vi "PacketToJSON.vi"(6 "StreamType(Raw)":T1, 8 "ErrorIn":errorcluster, 10 "Packet":T2={"ID"=0, "SamplesNr"=0, "Samples"=[], "MeasurementConfig"={"Frequency"=100, "Resolution[b]"=4, "AccelFSRange"=enum."+/-2g", "GyroFSRange"=enum."+/-250dps"}, "Comment"=""} {"MeasurementConfig"."Resolution[b]" min=4 max=16 step=1; "MeasurementConfig"."Frequency" min=1 max=10000000 step=1}, 11 "JSONIn":refnum<class "JSON Object.lvclass">) -> (0 "ErrorOut":errorcluster, 2 "JSONPacket":string, 3 "JSONOut":refnum<class "JSON Object.lvclass">)   [LabVIEW 2016]
doc: "Convert Packet to JSON. Return also JSONOut to combine with other JSON objects."
uses:
  FallSensor/Packet.ctl
  FallSensor/Sample.ctl
  FallSensor/Reading.ctl
  FallSensor/MeasurementConfig.ctl
  FallSensor/Measurement/AccelFSRange.ctl
  FallSensor/Measurement/GyroFSRange.ctl
  <vilib>/addons/JSON API/JSON Object/JSON Object.lvclass
  D:/Programy/National Instruments/LabVIEW 2016/vi.lib/addons/JSON API/JSON Value/JSON Value.lvclass
  JSONStreamType.ctl
  <vilib>/addons/JSON API/JSON Object/Set Object Item by name.vi
  <vilib>/addons/JSON API/JSON Value/Get as JSON string.vi
  <vilib>/addons/JSON API/JSON Scalar/JSON Scalar.lvclass
  <vilib>/addons/JSON API/JSON Array/JSON Array.lvclass
  <vilib>/addons/JSON API/JSON Scalar/Set U32.vi
  <vilib>/addons/JSON API/JSON Scalar/Set String.vi
  <vilib>/addons/JSON API/JSON Array/Set JSON Array.vi
  <vilib>/addons/JSON API/JSON Value/Get as JSON string (pretty).vi
  <vilib>/addons/JSON API/JSON Value/Get Item by name array.vi
  <vilib>/addons/JSON API/JSON Value/JSON Value.lvclass
  <vilib>/addons/JSON API/Get Polymorphic/JSON GetSet.lvlib
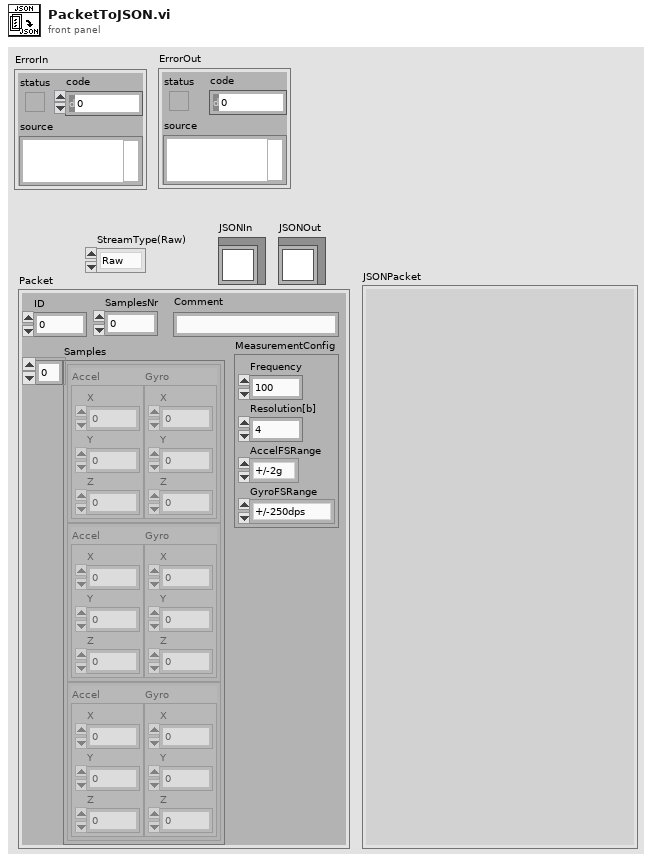
[diagram p1: front panel]
types:
  T1 = typedef "JSONStreamType.ctl" = enum16{"Raw", "Pretty"}
  T2 = typedef "Packet.ctl" = cluster{"ID":u32, "SamplesNr":u32, "Samples":T3[], "MeasurementConfig":T5, "Comment":string}
  T3 = typedef "Sample.ctl" = cluster{"Accel":T4, "Gyro":T4}
  T4 = typedef "Reading.ctl" = cluster{"X":i16, "Y":i16, "Z":i16}
  T5 = typedef "MeasurementConfig.ctl" = cluster{"Frequency":u32, "Resolution[b]":u32, "AccelFSRange":T6, "GyroFSRange":T7}
  T6 = typedef "AccelFSRange.ctl" = enum16{"+/-2g", "+/-4g", "+/-8g", "+/-16g"}
  T7 = typedef "GyroFSRange.ctl" = enum16{"+/-250dps", "+/-500dps", "+/-1000dps", "+/-2000dps"}
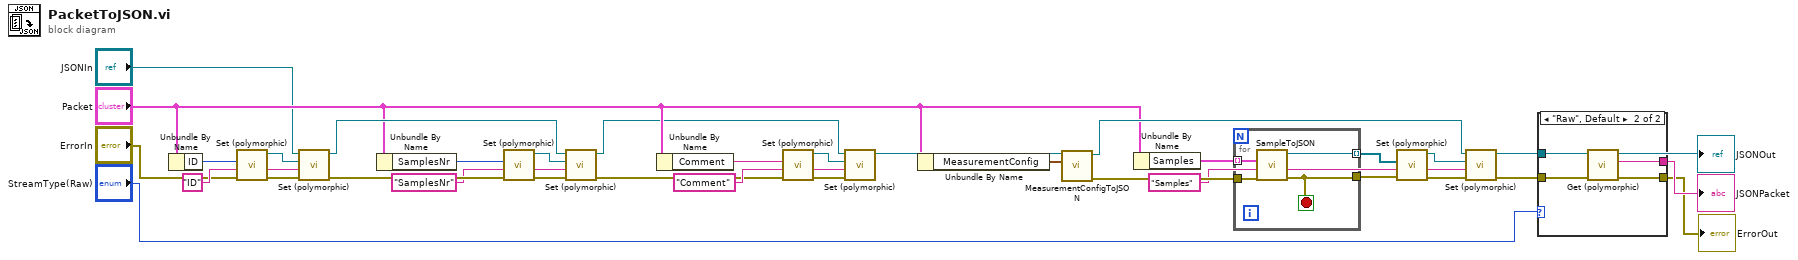
[diagram p0: block diagram]
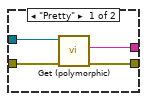
[diagram p2: hidden frame]
diagram:
  n1 = Unbundle By Name("Packet") -> ("ID"=w34:u32)
  n2 = call-poly <vilib>:"Set (polymorphic).vi"("error in (no error)"="ErrorIn", "Numeric"=w34) -> ("error out"=w29:errorcluster, "JSON Scalar out"=w33:refnum<class "JSON Scalar.lvclass">)  [unwired: 8 in]
  n3 = call-poly <vilib>:"Set (polymorphic).vi"("error in (no error)"=w29, "name"="ID", "Value"=w33, "JSON Object in"="JSONIn") -> ("error out"=w28:errorcluster, "JSON Object out"=w10:refnum<class "JSON Object.lvclass">)  [unwired: 5 in, 1 out]
  n4 = Unbundle By Name("Packet") -> ("SamplesNr"=w30:u32)
  n5 = call-poly <vilib>:"Set (polymorphic).vi"("error in (no error)"=w28, "Numeric"=w30) -> ("error out"=w25:errorcluster, "JSON Scalar out"=w31:refnum<class "JSON Scalar.lvclass">)  [unwired: 8 in]
  n6 = call-poly <vilib>:"Set (polymorphic).vi"("error in (no error)"=w25, "name"="SamplesNr", "Value"=w31, "JSON Object in"=w10) -> ("error out"=w8:errorcluster, "JSON Object out"=w6:refnum<class "JSON Object.lvclass">)  [unwired: 5 in, 1 out]
  n7 = Unbundle By Name("Packet") -> ("Comment"=w12:string)
  n8 = call-poly <vilib>:"Set (polymorphic).vi"("error in (no error)"=w8, "String"=w12) -> ("error out"=w14:errorcluster, "JSON Scalar out"=w11:refnum<class "JSON Scalar.lvclass">)  [unwired: 8 in]
  n9 = call-poly <vilib>:"Set (polymorphic).vi"("error in (no error)"=w14, "name"="Comment", "Value"=w11, "JSON Object in"=w6) -> ("JSON Object out"=w9:refnum<class "JSON Object.lvclass">)  [unwired: 5 in, 2 out]
  n10 = Unbundle By Name("Packet") -> ("MeasurementConfig"=w24:T5)
  n11 = call "MeasurementConfigToJSON.vi"("MeasurementConfig"=w24, "JSONIn"=w9) -> ("ErrorOut"=w22:errorcluster, "JSONOut"=w19:refnum<class "JSON Object.lvclass">)  [unwired: 7 in, 1 out]
  n12 = Unbundle By Name("Packet") -> ("Samples"=w15:T3[])
  n13 = for {
    tunnel: w22 -> [w38]
    tunnel: [w37] -> w18
    tunnel: [w36] -> w21 mode=indexing
    tunnel: w15 -> [w35] mode=indexing
    stop <- w37 stop-if-true
    n14 = call "SampleToJSON.vi"("ErrorIn"=w38, "Sample"=w35) -> ("ErrorOut"=w37:errorcluster, "JSONOut"=w36:refnum<class "JSON Object.lvclass">)  [unwired: 7 in, 1 out]
  }
  n15 = call-poly <vilib>:"Set (polymorphic).vi"("error in (no error)"=w18, "Array"=w21) -> ("error out"=w17:errorcluster, "JSON Array out"=w20:refnum<class "JSON Array.lvclass">)  [unwired: 8 in]
  n16 = call-poly <vilib>:"Set (polymorphic).vi"("error in (no error)"=w17, "name"="Samples", "Value"=w20, "JSON Object in"=w19) -> ("error out"=w4:errorcluster, "JSON Object out"=w3:refnum<class "JSON Object.lvclass">)  [unwired: 5 in, 1 out]
  "JSONOut" <- w3
  n17 = case shown="\"Raw\", Default" "StreamType(Raw)" {
    tunnel: [w42 w46] -> w23
    tunnel: w4 -> [w41 w45]
    tunnel: w3 -> [w40 w44]
    tunnel: [w39 w43] -> w2
    frame "Pretty" {
      n18 = call-poly <vilib>:"Get (polymorphic).vi"("error in (no error)"=w41, "JSON Value in"=w40) -> ("error out"=w39:errorcluster, "<JSON>"=w42:string)  [unwired: 8 in]
    }
    frame "Raw", Default {
      n19 = call-poly <vilib>:"Get (polymorphic).vi"("error in (no error)"=w45, "JSON Value in"=w44) -> ("error out"=w43:errorcluster, "<JSON>"=w46:string)  [unwired: 8 in]
    }
  }
  "ErrorOut" <- w2
  "JSONPacket" <- w23
